vi "_CallShell.vi"() -> ()   [LabVIEW 2019, in "lv-providershell-example3.lvlib"]
uses:
  lv-providershell-example3.lvlib
  Provider/ProviderClass.lvclass
  fd52217d-3635-4dc6-bc27-264ab1bf517b.vi
  fd52217d-3635-4dc6-bc27-264ab1bf517b.vi/e0920aba-d1db-49d7-8743-aa6dfbc522fe.vi
  fd52217d-3635-4dc6-bc27-264ab1bf517b.vi/c94616e3-ae69-46dd-a051-a73a6ee6adf1.vi
  fd52217d-3635-4dc6-bc27-264ab1bf517b.vi/20bc9264-8b73-4507-ade3-53cb14eaa897.vi
  fd52217d-3635-4dc6-bc27-264ab1bf517b.vi/0fb6571e-0d52-434d-97f3-83bf626383cd.vi
  <userlib>/_OpenG.lib/file/file.llb/File Exists__ogtk.vi
  <userlib>/_OpenG.lib/file/file.llb/File Exists - Scalar__ogtk.vi
  <userlib>/_OpenG.lib/file/file.llb/Strip Path Extension__ogtk.vi
  <userlib>/_OpenG.lib/file/file.llb/Strip Path Extension - Path__ogtk.vi
  <vilib>/Utility/LVLibp/Get Exported File List.vi
  <vilib>/Utility/LVClass/Get LV Class Default Value.vi
  _Support/__Wait(ms) If Input Valid.vi
  <vilib>/Utility/libraryn.llb/Check if File or Folder Exists.vi
  ClassProviderShellHelper/__Safely Recursive File List.vi
  <userlib>/_OpenG.lib/file/file.llb/Compare Two Paths__ogtk.vi
  <userlib>/_OpenG.lib/file/file.llb/Compare Two Paths - Scalar__ogtk.vi
  <userlib>/_OpenG.lib/file/file.llb/Build Path__ogtk.vi
  <userlib>/_OpenG.lib/file/file.llb/Build Path - File Names Array__ogtk.vi
panel:
  out "Array 2":string[](array[string])
  out "Array":bool[](array[boolean])
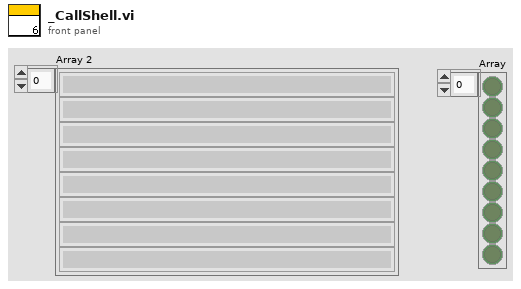
[diagram p1: front panel]
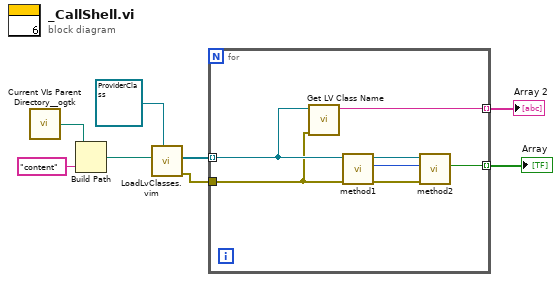
[diagram p0: block diagram]
diagram:
  n1 = call <userlib>:"Current VIs Parent Directory__ogtk.vi"() -> ("Parent Directory (+ Relative)"=w7:path)  [unwired: 5 in]
  n2 = Build Path(base path=w7, name or relative path="content") -> (appended path=w5:path)
  n3 = call "LoadLvClasses.vim"("ClassType"=refnum<class "ProviderClass.lvclass"> refnum ("lv-providershell-example3.lvlib:ProviderClass.lvclass"), "Path"=w5) -> ("error out"=w2:errorcluster, "Loaded Classes"=w4:refnum<class "ProviderClass.lvclass">[])  [unwired: 8 in]
  n4 = for {
    tunnel: w4 -> [w11] mode=indexing
    tunnel: [w12] -> w3 mode=indexing
    tunnel: w2 -> [w10]
    tunnel: [w9] -> w1 mode=indexing
    n5 = call <vilib>:"Get LV Class Name.vi"("error in (no error)"=w10, "object"=w11) -> ("class name"=w9:string)  [unwired: 8 in, 1 out]
    n6 = call-dynamic "method1.vi"("error in (no error)"=w10, "ProviderClass in"=w11) -> ("error out"=w13:errorcluster, "RefNum"=w14:i32, "ProviderClass out"=w15:refnum<class "ProviderClass.lvclass">)  [unwired: 7 in]
    n7 = call-dynamic "method2.vi"("error in (no error)"=w13, "RefNum"=w14, "ProviderClass in"=w15) -> ("Boolean"=w12:bool)  [unwired: 6 in, 2 out]
  }
  "Array" <- w3
  "Array 2" <- w1
